vi "Log String.vi"(6 "String":string, 8 "error in (no error)":errorcluster, 11 "String Control Sink in":refnum<class "String Control Sink.lvclass">) -> (0 "error out":errorcluster, 3 "String Control Sink out":refnum<class "String Control Sink.lvclass">)   [LabVIEW 2016, in "Stream Log.lvlib" / "String Control Sink.lvclass"]
doc: "--\nCopyright © 2017 Composed SystemsI All rights reserved.\n\nAuthor: Jon McBee <jon.mcbee@composed.io>\n\nThis library is provided \"AS IS\" ,WITHOUT WARRANTIES OR\nCONDITIONS OF ANY KIND, either express or implied.\n\nComposed Systems -- composed.io\n\nStream 0.0.1.1\nJon McBee - Composed Systems\nCopyright (c) 2017, Composed Systems"
uses:
  <userlib>/Composed Systems/Stream/Log/String Control Sink/String Control Sink.lvclass
  <userlib>/Composed Systems/Stream/Log/String Control Sink/String Control Sink.lvclass/String Control Sink.ctl
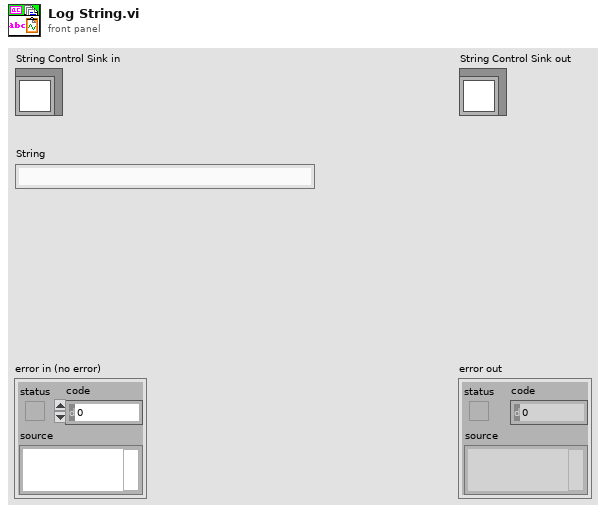
[diagram p1: front panel]
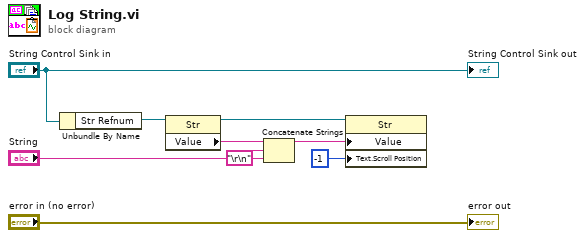
[diagram p0: block diagram]
diagram:
  n1 = Unbundle By Name("String Control Sink in") -> ("Str Refnum"=w8:refnum<vi>)
  n2 = property class="Str"(reference=w8) -> (reference out=w4:refnum<vi>, "Value"=w7:string)  [unwired: 1 in, 1 out]
  n3 = Concatenate Strings(w7, "String", "\r\n") -> (w3:string)
  n4 = property class="Str"(reference=w4, "Value"=w3, "Text.Scroll Position"=-1) -> ()  [unwired: 1 in, 2 out]
  "error out" <- "error in (no error)"
  "String Control Sink out" <- "String Control Sink in"
